vi "RSNRPZ Configure Source Gamma Corr.vi"(6 "Magnitude (1.0)":dbl=1.0 format="%.2p", 7 "Phase (0.0 deg)":dbl format="%.2p", 8 "error in (no error)":errorcluster, 9 "Source Gamma Correction (F: Off)":bool, 10 "Channel (1)":i32=1, 11 "VISA session":refnum<visa-resource-name> caption="VISA resource name") -> (0 "error out":errorcluster, 3 "dup VISA session":refnum<visa-resource-name> caption="VISA resource name")   [LabVIEW 2010]
doc: "This VI sets the parameters of the reflection coefficient for measured-value correction.\n\nRemote-control command(s):\nSENSe[1..4]:SGAMma\nSENSe[1..4]:SGAMma:PHASe\nSENSe[1..4]:SGAMma:CORRection:STATe ON | OFF"
uses:
  rsnrpz_32.dll
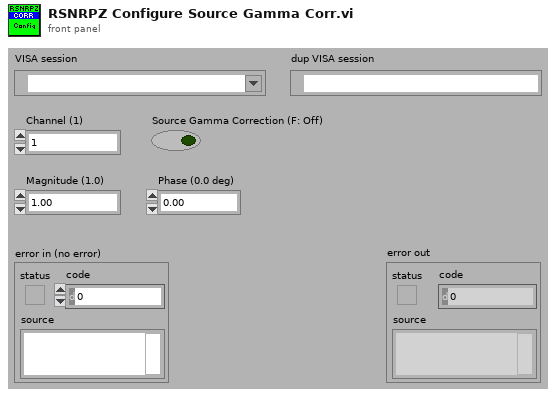
[diagram p1: front panel]
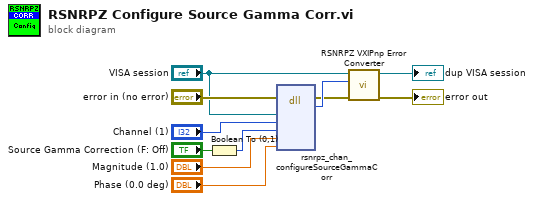
[diagram p0: block diagram]
diagram:
  n1 = Boolean To (0,1)(Boolean="Source Gamma Correction (F: Off)") -> (0, 1=w8:i16)
  n2 = dll-call lib="rsnrpz_32.dll" fn="rsnrpz_chan_configureSourceGammaCorr"(error in="error in (no error)", "VISA Session"="VISA session", "Channel"="Channel (1)", "Source Gamma Correction"=w8, "Magnitude"="Magnitude (1.0)", "Phase"="Phase (0.0 deg)") -> (error out=w5:errorcluster, "Status"=w10:i32)  [unwired: 7 in, 1 out]
  n3 = call <instrlib>:"RSNRPZ VXIPnp Error Converter.vi"("error in"=w5, "VXIPnp error code"=w10, "VISA session"="VISA session") -> ("error out"=→"error out":errorcluster, "dup VISA session"=→"dup VISA session":refnum<visa-resource-name>)  [unwired: 7 in]
